vi "Need Chop.vi"(11 "bin":cluster{"lower limit":dbl, "upper limit":dbl}) -> (3 "chop?":bool)   [LabVIEW 2017, in "NI_AALPro.lvlib"]
uses:
  <vilib>/Analysis/NI_AALPro.lvlib
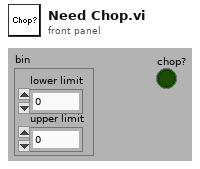
[diagram p1: front panel]
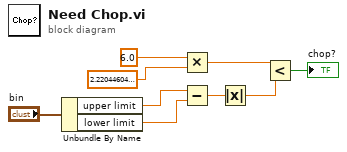
[diagram p0: block diagram]
diagram:
  n1 = Unbundle By Name("bin") -> ("upper limit"=w4:dbl, "lower limit"=w3:dbl)
  n2 = Multiply(x=6.0, y=2.220446049250313e-16 ("x^y")) -> (x*y=w5:dbl)
  n3 = Subtract(x=w4, y=w3) -> (x-y=w9:dbl)
  n4 = Absolute Value(x=w9) -> (abs(x)=w6:dbl)
  n5 = Less?(x=w5, y=w6) -> (x < y?=→"chop?":bool)
